vi "PowerSupply SelfTest.vi"(8 "error in":errorcluster) -> (0 "error out":errorcluster, 2 "Report Text":string, 3 "OK":bool)   [LabVIEW 2023, in "LTT_TeststandSteptypes.lvlib"]
uses:
  LTT_TeststandSteptypes.lvlib
  HardwareAbstractionLayer_LVOOP/Teststand/Teststand.lvclass
  HardwareAbstractionLayer_LVOOP/Database/Database.lvclass
  <userlib>/_OpenG.lib/error/error.llb/openg_error.lvlib
panel:
  out "IP Status":string
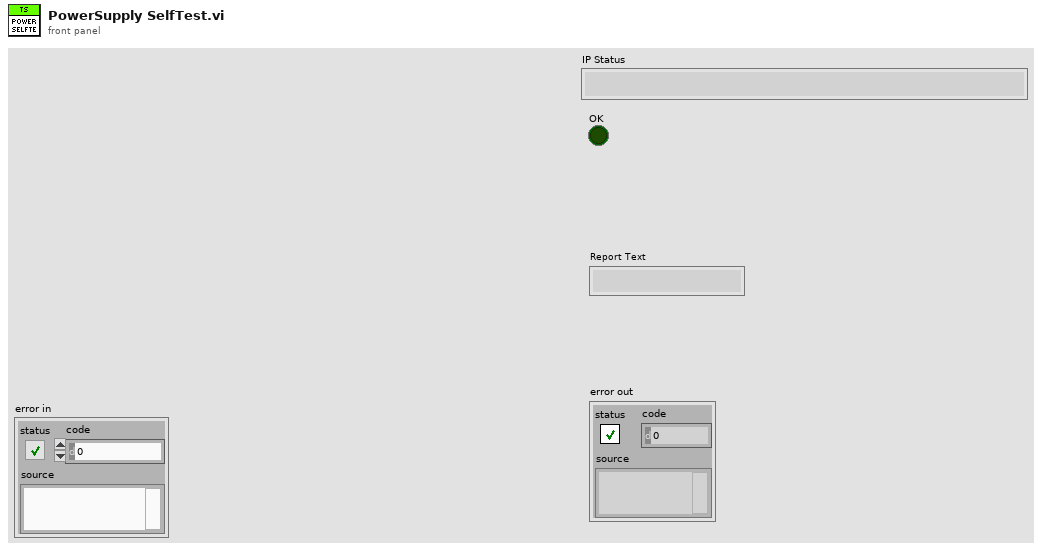
[diagram p1: front panel]
types:
  T1 = typedef "HardwareAbstractionLayer_LVOOP.lvlib/Teststand.lvclass/Teststand Status Control.ctl" = cluster{"Terminating or Aborting":bool, "Stop":bool, "Socket Count":i16, "Selected Sockets":i16[]}
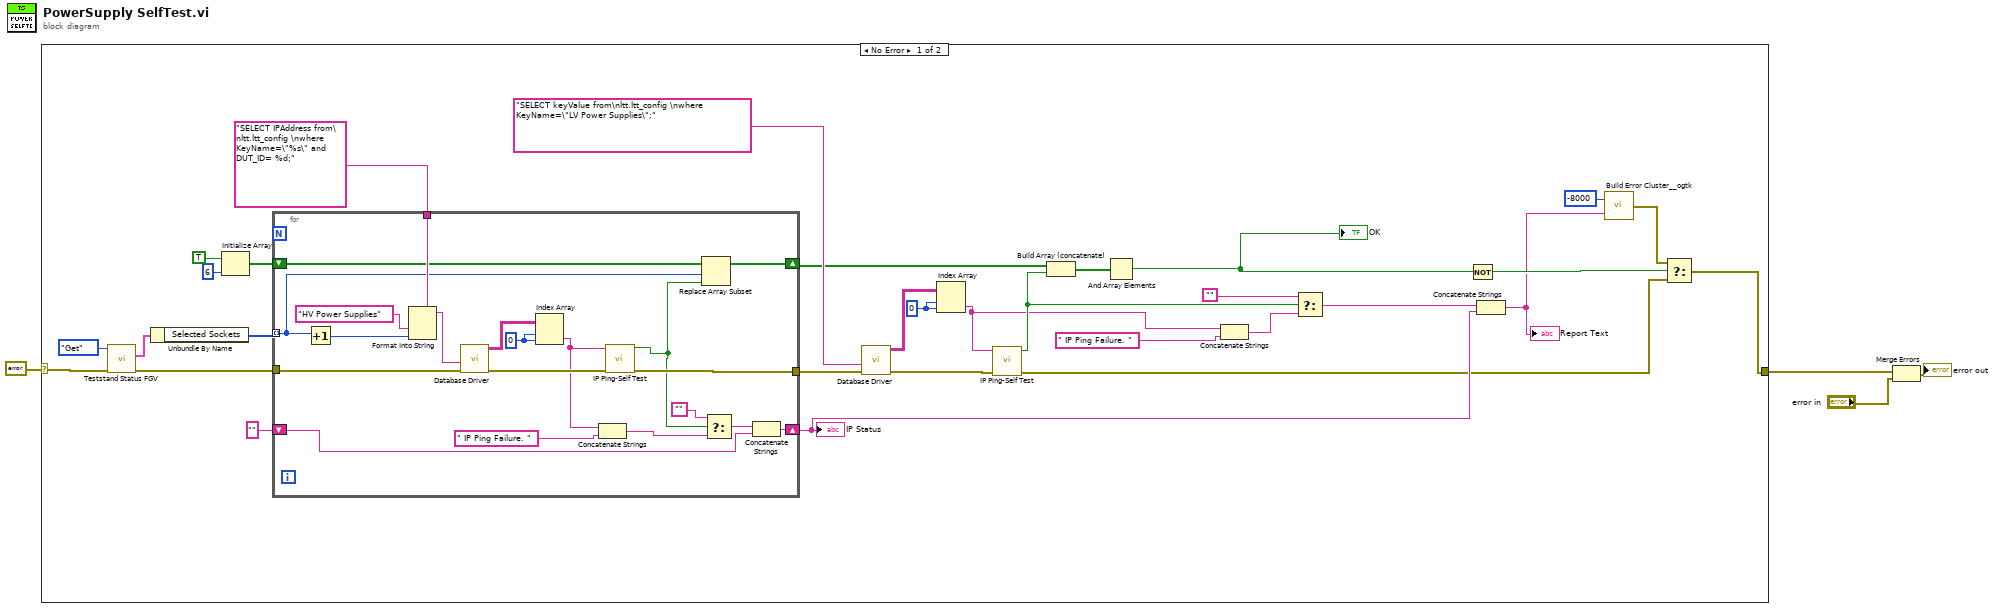
[diagram p0: block diagram]
diagram:
  n1 = case shown="No Error" errorcluster {"status"=FALSE, "code"=0, "source"=""} ("error IO") {
    selector: errorcluster {"status"=FALSE, "code"=0, "source"=""} ("error IO") -> [w12 w56]
    tunnel: [w8 w56] -> w4
    frame No Error {
      w31 = 0 ("index (row)")
      n2 = call "Teststand Status FGV.vi"("error in"=w12, "Option"=enum16{"Set", "Get"}."Get") -> ("error out"=w32:errorcluster, "Teststand Status Out"=w34:T1)  [unwired: 8 in]
      n3 = Unbundle By Name(w34) -> ("Selected Sockets"=w21:i16[])
      n4 = Initialize Array(TRUE, 6 ("dimension size")) -> (w24:bool[])
      n5 = for {
        tunnel: "SELECT IPAddress from\nltt.ltt_config \nwhere KeyName=\"%s\" and DUT_ID= %d;" -> [w54]
        tunnel: w32 -> [w53]
        tunnel: [w38] -> w29
        shift-right: [w48] -> w13
        shift-left: "" -> [w47]
        shift-right: [w41] -> w23
        shift-left: w24 -> [w42]
        tunnel: w21 -> [w40] mode=indexing
        w51 = 0 ("index (row)")
        n6 = Increment(x=w40) -> (x+1=w46:i16)
        n7 = Format Into String(format string=w54, "HV Power Supplies", w46) -> (resulting string=w44:string)  [unwired: 2 in, 1 out]
        n8 = call "Database Driver.vi"("error in"=w53, "SQL query"=w44) -> ("error out"=w39:errorcluster, "data"=w52:string[][])  [unwired: 6 in, 2 out]
        n9 = Index Array(array=w52, index (row)=w51, index (col)=w51) -> (element=w37:string)
        n10 = Concatenate Strings(w37, " IP Ping Failure. ") -> (w45:string)
        n11 = call "IP Ping-Self Test.vi"("error in (no error)"=w39, "IP/Address"=w37) -> ("error out"=w38:errorcluster, "Sucessful?"=w36:bool)  [unwired: 8 in]
        n12 = Replace Array Subset(array=w42, new element=w36, index=w40) -> (w41:bool[])
        n13 = Select(t="", s=w36, f=w45) -> (s? t:f=w49:string)
        n14 = Concatenate Strings(w49, w47) -> (w48:string)
      }
      "IP Status" <- w13
      n15 = call "Database Driver.vi"("error in"=w29, "SQL query"="SELECT keyValue from\nltt.ltt_config \nwhere KeyName=\"LV Power Supplies\";") -> ("error out"=w20:errorcluster, "data"=w30:string[][])  [unwired: 6 in, 2 out]
      n16 = Index Array(array=w30, index (row)=w31, index (col)=w31) -> (element=w16:string)
      n17 = call "IP Ping-Self Test.vi"("error in (no error)"=w20, "IP/Address"=w16) -> ("error out"=w9:errorcluster, "Sucessful?"=w19:bool)  [unwired: 8 in]
      n18 = Build Array (concatenate)(w23, w19) -> (w22:bool[])
      n19 = And Array Elements(Boolean array=w22) -> (logical AND=w7:bool)
      "OK" <- w7
      n20 = Concatenate Strings(w16, " IP Ping Failure. ") -> (w15:string)
      n21 = Select(t="", s=w19, f=w15) -> (s? t:f=w14:string)
      n22 = Not(x=w7) -> (.not. x?=w6:bool)
      n23 = Concatenate Strings(w14, w13) -> (w5:string)
      "Report Text" <- w5
      n24 = call <userlib>:"Build Error Cluster__ogtk.vi"("String to Prepend to source (\"\")"=w5, "code"=-8000) -> ("error out"=w11:errorcluster)
      n25 = Select(t=w11, s=w6, f=w9) -> (s? t:f=w8:errorcluster)
    }
    frame Error {
    }
  }
  n26 = Merge Errors(w4, "error in") -> (→"error out":errorcluster)
